vi "ArduinoMultiChannelTest .vi"() -> ()   [LabVIEW 2019]
uses:
  <vilib>/Instr/_visa.llb/VISA Configure Serial Port (Instr).vi
panel:
  out "Waveform Chart 4":dbl(graph)
  out "Waveform Chart 3":dbl(graph)
  in  "Baud Rate 2":u32=9600
  in  "COM Port 2":refnum<visa-resource-name>
  in  "Stop Button":bool
  out "Available?":bool
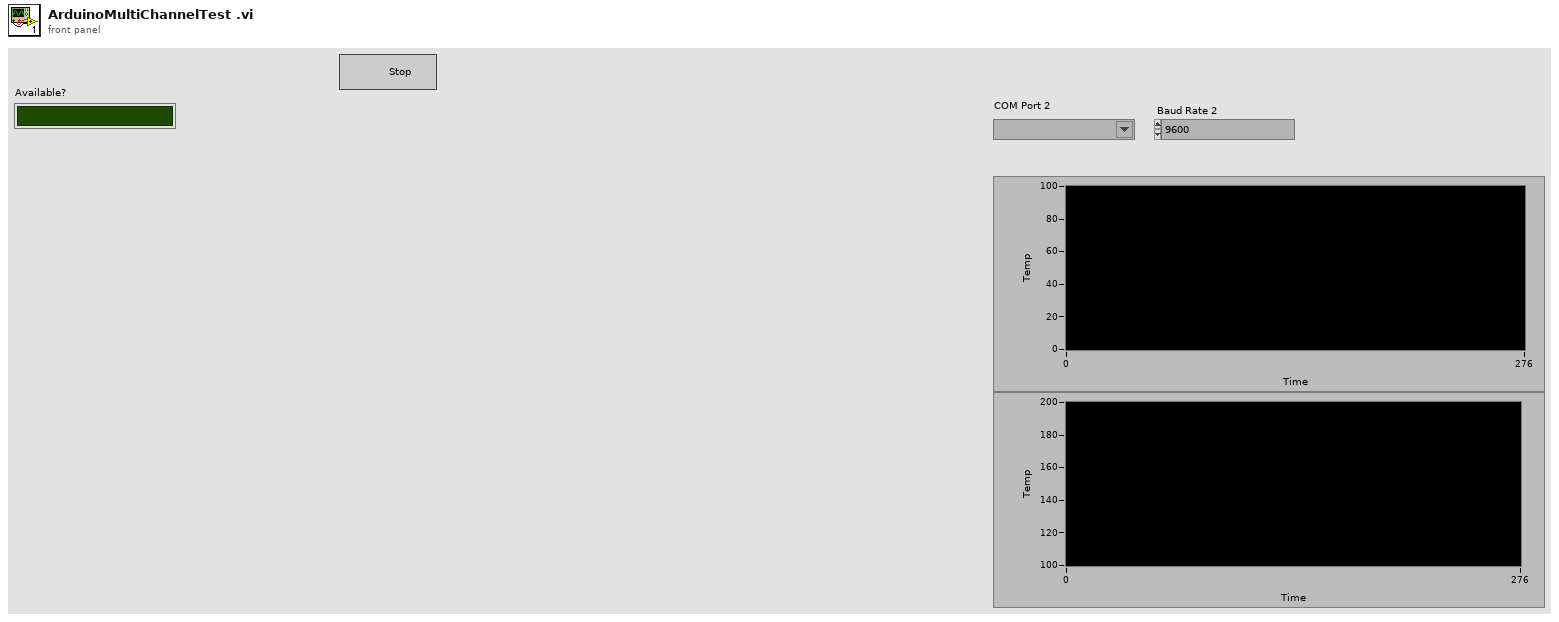
[diagram p1: front panel]
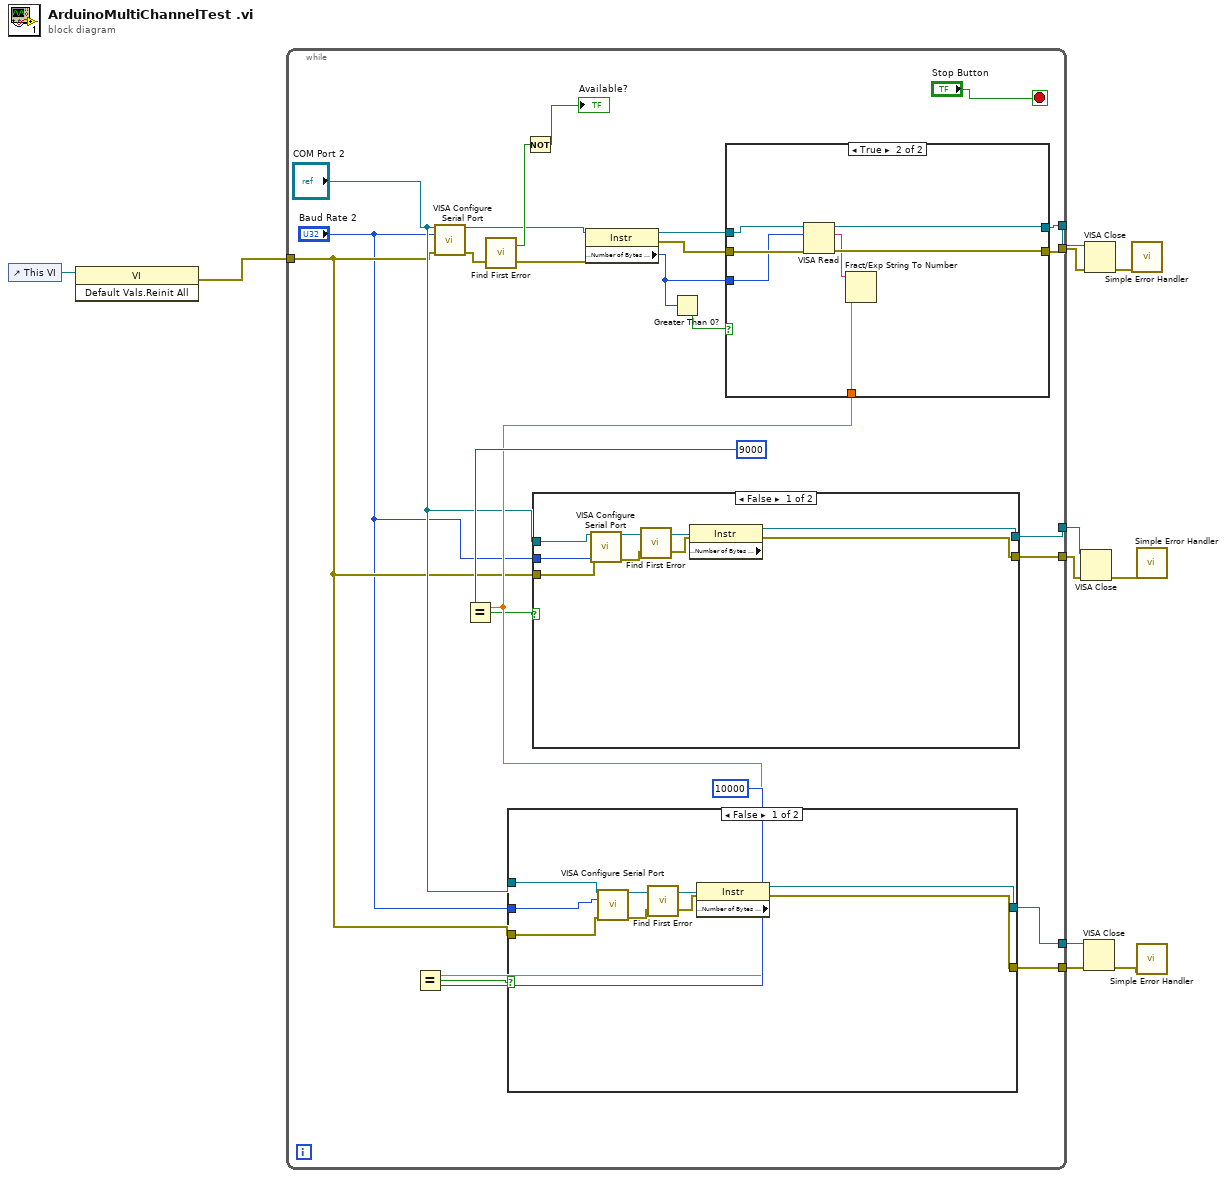
[diagram p0: block diagram]
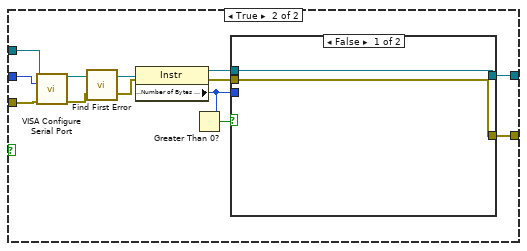
[diagram p2: hidden frame]
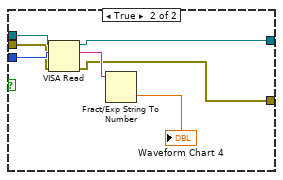
[diagram p3: hidden frame]
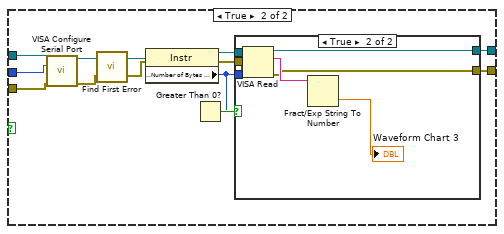
[diagram p4: hidden frame]
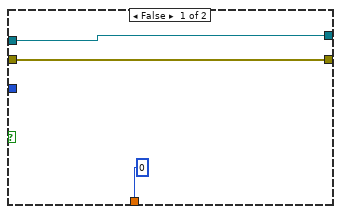
[diagram p6: hidden frame]
diagram:
  n1 = control-ref of="This VI"() -> (w7:refnum<vi>)
  n2 = invoke class="VI" method="Default Vals.Reinit All"(reference=w7) -> (error out=w8:errorcluster)  [unwired: 2 in, 2 out]
  n3 = while {
    tunnel: [w32] -> w10
    tunnel: [w31] -> w11
    tunnel: w8 -> [w15]
    tunnel: [w21] -> w5
    tunnel: [w22] -> w4
    tunnel: [w19] -> w2
    tunnel: [w18] -> w1
    stop <- "Stop Button" stop-if-true
    n4 = call-poly "VISA Configure Serial Port"("VISA resource name"="COM Port 2", "baud rate (9600)"="Baud Rate 2", "error in (no error)"=w15) -> ("VISA resource name out"=w24:refnum<visa-resource-name>, "error out"=w28:errorcluster)  [unwired: 11 in]
    n5 = call <vilib>:"Find First Error.vi"("error in (no error)"=w28) -> ("error out"=w25:errorcluster, "error?"=w27:bool)  [unwired: 3 in]
    n6 = Not(x=w27) -> (.not. x?=→"Available?":bool)
    n7 = property class="Instr"(reference=w24, error in=w25) -> (reference out=w33:refnum<visa-resource-name>, error out=w34:errorcluster, "Serial Settings:Number of Bytes at Serial Port"=w30:u32)
    n8 = Greater Than 0?(x=w30) -> (x > 0?=w35:bool)
    n9 = case shown="True" w35 {
      tunnel: w33 -> [w96 w103]
      tunnel: w34 -> [w95 w101]
      tunnel: [w96 w102] -> w32
      tunnel: [w95 w100] -> w31
      tunnel: w30 -> [_ w99]
      tunnel: [0 w97] -> w17
      frame False {
      }
      frame True {
        n10 = VISA Read(VISA resource name=w103, byte count=w99, error in (no error)=w101) -> (VISA resource name out=w102:refnum<visa-resource-name>, read buffer=w98:string, error out=w100:errorcluster)  [unwired: 1 out]
        n11 = Fract/Exp String To Number(string=w98) -> (number=w97:dbl)  [unwired: 3 in, 1 out]
      }
    }
    n12 = Equal?(x=w17, y=10000) -> (x = y?=w13:bool)
    n13 = Equal?(x=w17, y=9000) -> (x = y?=w12:bool)
    n14 = case shown="False" w13 {
      tunnel: "COM Port 2" -> [w40 w48]
      tunnel: w15 -> [w38 w49]
      tunnel: [w37 w55] -> w19
      tunnel: [w36 w54] -> w18
      tunnel: "Baud Rate 2" -> [w39 w50]
      frame False {
        n15 = call-poly "VISA Configure Serial Port"("VISA resource name"=w40, "baud rate (9600)"=w39, "error in (no error)"=w38) -> ("VISA resource name out"=w41:refnum<visa-resource-name>, "error out"=w43:errorcluster)  [unwired: 11 in]
        n16 = call <vilib>:"Find First Error.vi"("error in (no error)"=w43) -> ("error out"=w42:errorcluster)  [unwired: 3 in, 1 out]
        n17 = property class="Instr" props=["Serial Settings:Number of Bytes at Serial Port"](reference=w41, error in=w42) -> (reference out=w37:refnum<visa-resource-name>, error out=w36:errorcluster)  [unwired: 1 out]
      }
      frame True {
        n18 = call-poly "VISA Configure Serial Port"("VISA resource name"=w48, "baud rate (9600)"=w50, "error in (no error)"=w49) -> ("VISA resource name out"=w53:refnum<visa-resource-name>, "error out"=w51:errorcluster)  [unwired: 11 in]
        n19 = call <vilib>:"Find First Error.vi"("error in (no error)"=w51) -> ("error out"=w52:errorcluster)  [unwired: 3 in, 1 out]
        n20 = property class="Instr"(reference=w53, error in=w52) -> (reference out=w47:refnum<visa-resource-name>, error out=w46:errorcluster, "Serial Settings:Number of Bytes at Serial Port"=w44:u32)
        n21 = Greater Than 0?(x=w44) -> (x > 0?=w45:bool)
        n22 = case shown="False" w45 {
          tunnel: [w57 w62] -> w55
          tunnel: [w56 w61] -> w54
          tunnel: w47 -> [w57 w60]
          tunnel: w44 -> [_ w59]
          tunnel: w46 -> [w56 w58]
          frame False {
          }
          frame True {
            n23 = VISA Read(VISA resource name=w60, byte count=w59, error in (no error)=w58) -> (VISA resource name out=w62:refnum<visa-resource-name>, read buffer=w64:string, error out=w61:errorcluster)  [unwired: 1 out]
            n24 = Fract/Exp String To Number(string=w64) -> (number=→"Waveform Chart 4":dbl)  [unwired: 3 in, 1 out]
          }
        }
      }
    }
    n25 = case shown="False" w12 {
      tunnel: w15 -> [w67 w80]
      tunnel: "COM Port 2" -> [w69 w81]
      tunnel: [w66 w84] -> w22
      tunnel: [w65 w83] -> w21
      tunnel: "Baud Rate 2" -> [w68 w82]
      frame False {
        n26 = call-poly "VISA Configure Serial Port"("VISA resource name"=w69, "baud rate (9600)"=w68, "error in (no error)"=w67) -> ("VISA resource name out"=w72:refnum<visa-resource-name>, "error out"=w70:errorcluster)  [unwired: 11 in]
        n27 = call <vilib>:"Find First Error.vi"("error in (no error)"=w70) -> ("error out"=w71:errorcluster)  [unwired: 3 in, 1 out]
        n28 = property class="Instr" props=["Serial Settings:Number of Bytes at Serial Port"](reference=w72, error in=w71) -> (reference out=w66:refnum<visa-resource-name>, error out=w65:errorcluster)  [unwired: 1 out]
      }
      frame True {
        n29 = call-poly "VISA Configure Serial Port"("VISA resource name"=w81, "baud rate (9600)"=w82, "error in (no error)"=w80) -> ("VISA resource name out"=w77:refnum<visa-resource-name>, "error out"=w79:errorcluster)  [unwired: 11 in]
        n30 = call <vilib>:"Find First Error.vi"("error in (no error)"=w79) -> ("error out"=w78:errorcluster)  [unwired: 3 in, 1 out]
        n31 = property class="Instr"(reference=w77, error in=w78) -> (reference out=w76:refnum<visa-resource-name>, error out=w75:errorcluster, "Serial Settings:Number of Bytes at Serial Port"=w73:u32)
        n32 = Greater Than 0?(x=w73) -> (x > 0?=w74:bool)
        n33 = case shown="True" w74 {
          tunnel: [w86 w91] -> w84
          tunnel: [w85 w90] -> w83
          tunnel: w76 -> [w86 w89]
          tunnel: w73 -> [_ w88]
          tunnel: w75 -> [w85 w87]
          frame False {
          }
          frame True {
            n34 = VISA Read(VISA resource name=w89, byte count=w88, error in (no error)=w87) -> (VISA resource name out=w91:refnum<visa-resource-name>, read buffer=w93:string, error out=w90:errorcluster)  [unwired: 1 out]
            n35 = Fract/Exp String To Number(string=w93) -> (number=→"Waveform Chart 3":dbl)  [unwired: 3 in, 1 out]
          }
        }
      }
    }
  }
  n36 = VISA Close(VISA resource name=w4, error in (no error)=w5) -> (error out=w6:errorcluster)
  n37 = VISA Close(VISA resource name=w2, error in (no error)=w1) -> (error out=w3:errorcluster)
  n38 = VISA Close(VISA resource name=w10, error in (no error)=w11) -> (error out=w9:errorcluster)
  n39 = call <vilib>:"Simple Error Handler.vi"("error in (no error)"=w9) -> ()  [unwired: 4 in, 5 out]
  n40 = call <vilib>:"Simple Error Handler.vi"("error in (no error)"=w6) -> ()  [unwired: 4 in, 5 out]
  n41 = call <vilib>:"Simple Error Handler.vi"("error in (no error)"=w3) -> ()  [unwired: 4 in, 5 out]
